vi "Get Alias.vi"(8 "error in (no error)":errorcluster, 11 "Instrument List Data in":refnum<class "Instrument List Data.lvclass">) -> (0 "error out":errorcluster, 2 "Alias":string, 3 "Instrument List Data out":refnum<class "Instrument List Data.lvclass">)   [LabVIEW 2020, in "Instrument Handler.lvlib" / "Instrument List Data.lvclass"]
doc: "Return the Alias of the Data class.\n\nThis implementation returns 'Instrument List'."
uses:
  Instrument List Data.lvclass
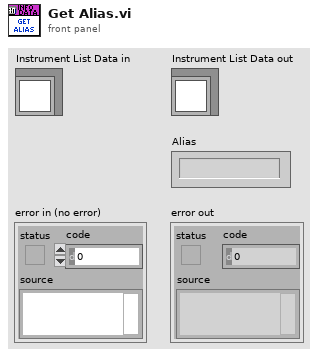
[diagram p1: front panel]
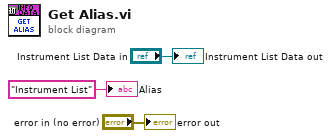
[diagram p0: block diagram]
diagram:
  "error out" <- "error in (no error)"
  "Instrument List Data out" <- "Instrument List Data in"
  "Alias" <- "Instrument List" ("Alias")
